vi "Luminosity to ASCII.vi"(11 "Luminosity":u8) -> (3 "ASCII Char":string)   [LabVIEW 2018, in "Colour Lab.lvlib"]
uses:
  Colour Lab.lvlib
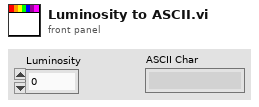
[diagram p1: front panel]
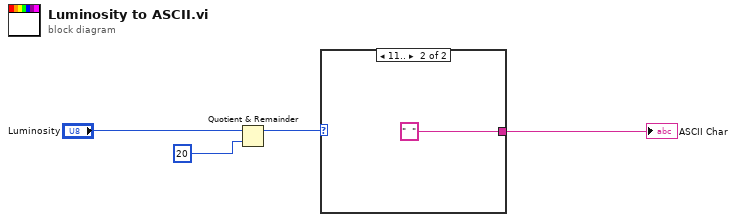
[diagram p0: block diagram]
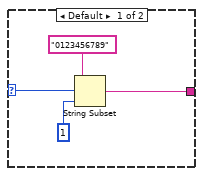
[diagram p2: hidden frame]
diagram:
  n1 = Quotient & Remainder(x="Luminosity", y=20 ("length")) -> (x-y*floor(x/y)=w1:i32)  [unwired: 1 out]
  n2 = case shown="11.." w1 {
    selector: w1 -> [w5 _]
    tunnel: [w8 "  "] -> w4
    frame Default {
      n3 = String Subset(string="0123456789", offset (0)=w5, length (rest)=1 ("length (rest)")) -> (substring=w8:string)
    }
    frame 11.. {
    }
  }
  "ASCII Char" <- w4
